vi "Axis Property to Array.vi"(11 "Axis Property In":T2) -> (3 "Axis Property Array Out":T1[](array[typedef]))   [LabVIEW 2020, in "3D Plot.lvclass"]
uses:
  3D Plot.lvclass
  Axis Property.ctl
  Caption Property.ctl
  Label Property.ctl
  Range Property.ctl
  Range Clusters.ctl
  Grid Property.ctl
  Tick Property.ctl
  Axis Property Array Element.ctl
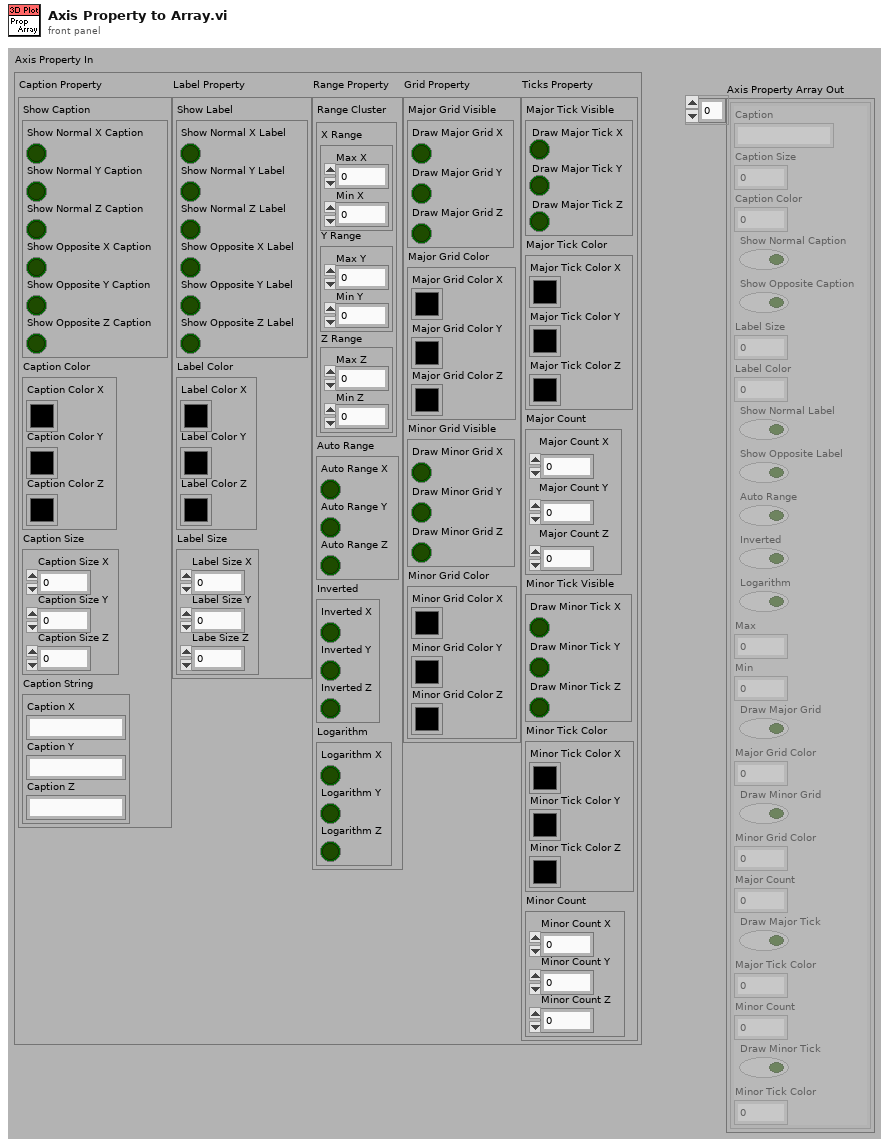
[diagram p1: front panel]
types:
  T1 = typedef "3D Plot.lvclass/Axis Property Array Element.ctl" = cluster{"Caption":string, "Caption Size":u16, "Caption Color":u32, "Show Normal Caption":bool, "Show Opposite Caption":bool, "Label Size":u16, "Label Color":u32, "Show Normal Label":bool, "Show Opposite Label":bool, "Auto Range":bool, "Inverted":bool, "Logarithm":bool, "Max":sgl, "Min":sgl, "Draw Major Grid":bool, "Major Grid Color":u32, "Draw Minor Grid":bool, "Minor Grid Color":u32, "Major Count":u16, "Draw Major Tick":bool, "Major Tick Color":u32, "Minor Count":u16, "Draw Minor Tick":bool, "Minor Tick Color":u32}
  T2 = typedef "3D Plot.lvclass/Axis Property.ctl" = cluster{"Caption Property":T3, "Label Property":T4, "Range Property":T5, "Grid Property":T7, "Ticks Property":T8}
  T3 = typedef "3D Plot.lvclass/Caption Property.ctl" = cluster{"Show Caption":cluster{"Show Normal X Caption":bool, "Show Normal Y Caption":bool, "Show Normal Z Caption":bool, "Show Opposite X Caption":bool, "Show Opposite Y Caption":bool, "Show Opposite Z Caption":bool}, "Caption Color":cluster{"Caption Color X":u32, "Caption Color Y":u32, "Caption Color Z":u32}, "Caption Size":cluster{"Caption Size X":u16, "Caption Size Y":u16, "Caption Size Z":u16}, "Caption String":cluster{"Caption X":string, "Caption Y":string, "Caption Z ":string}}
  T4 = typedef "3D Plot.lvclass/Label Property.ctl" = cluster{"Show Label":cluster{"Show Normal X Label":bool, "Show Normal Y Label":bool, "Show Normal Z Label":bool, "Show Opposite X Label":bool, "Show Opposite Y Label":bool, "Show Opposite Z Label":bool}, "Label Color":cluster{"Label Color X":u32, "Label Color Y":u32, "Label Color Z":u32}, "Label Size":cluster{"Label Size X":u16, "Label Size Y":u16, "Labe Size Z":u16}}
  T5 = typedef "3D Plot.lvclass/Range Property.ctl" = cluster{"Range Cluster":T6, "Auto Range":cluster{"Auto Range X":bool, "Auto Range Y":bool, "Auto Range Z":bool}, "Inverted":cluster{"Inverted X":bool, "Inverted Y":bool, "Inverted Z":bool}, "Logarithm":cluster{"Logarithm X":bool, "Logarithm Y":bool, "Logarithm Z":bool}}
  T6 = typedef "3D Plot.lvclass/Range Clusters.ctl" = cluster{"X Range":cluster{"Max X":sgl, "Min X":sgl}, "Y Range":cluster{"Max Y":sgl, "Min Y":sgl}, "Z Range":cluster{"Max Z":sgl, "Min Z":sgl}}
  T7 = typedef "3D Plot.lvclass/Grid Property.ctl" = cluster{"Major Grid Visible":cluster{"Draw Major Grid X":bool, "Draw Major Grid Y":bool, "Draw Major Grid Z":bool}, "Major Grid Color":cluster{"Major Grid Color X":u32, "Major Grid Color Y":u32, "Major Grid Color Z":u32}, "Minor Grid Visible":cluster{"Draw Minor Grid X":bool, "Draw Minor Grid Y":bool, "Draw Minor Grid Z":bool}, "Minor Grid Color":cluster{"Minor Grid Color X":u32, "Minor Grid Color Y":u32, "Minor Grid Color Z":u32}}
  T8 = typedef "3D Plot.lvclass/Tick Property.ctl" = cluster{"Major Tick Visible":cluster{"Draw Major Tick X":bool, "Draw Major Tick Y":bool, "Draw Major Tick Z":bool}, "Major Tick Color":cluster{"Major Tick Color X":u32, "Major Tick Color Y":u32, "Major Tick Color Z":u32}, "Major Count":cluster{"Major Count X":u16, "Major Count Y":u16, "Major Count Z":u16}, "Minor Tick Visible":cluster{"Draw Minor Tick X":bool, "Draw Minor Tick Y":bool, "Draw Minor Tick Z":bool}, "Minor Tick Color":cluster{"Minor Tick Color X":u32, "Minor Tick Color Y":u32, "Minor Tick Color Z":u32}, "Minor Count":cluster{"Minor Count X":u16, "Minor Count Y":u16, "Minor Count Z":u16}}
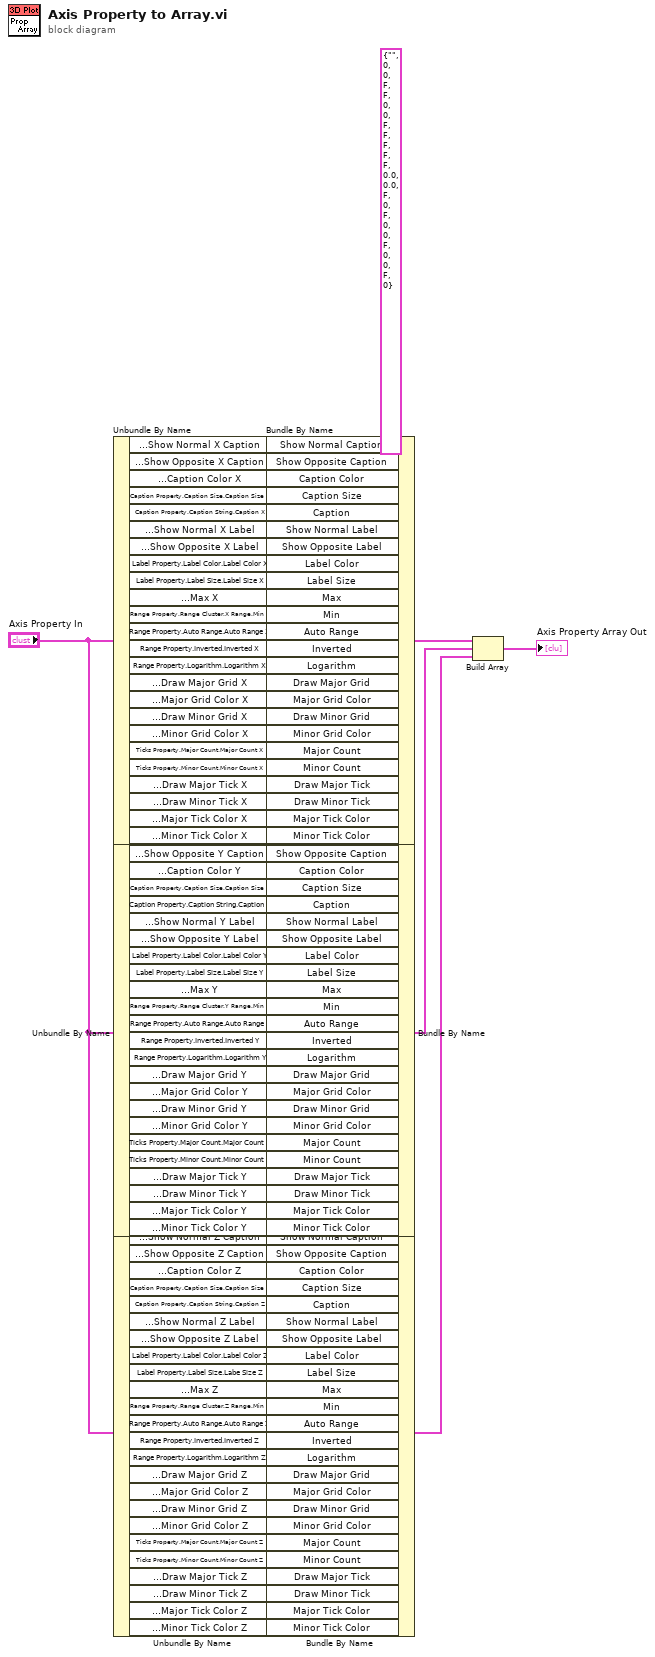
[diagram p0: block diagram]
diagram:
  w6 = T1 {"Caption"="", "Caption Size"=0, "Caption Color"=0, "Show Normal Caption"=FALSE, "Show Opposite Caption"=FALSE, "Label Size"=0, "Label Color"=0, "Show Normal Label"=FALSE, "Show Opposite Label"=FALSE, "Auto Range"=FALSE, "Inverted"=FALSE, "Logarithm"=FALSE, "Max"=0.0, "Min"=0.0, "Draw Major Grid"=FALSE, "Major Grid Color"=0, "Draw Minor Grid"=FALSE, "Minor Grid Color"=0, "Major Count"=0, "Draw Major Tick"=FALSE, "Major Tick Color"=0, "Minor Count"=0, "Draw Minor Tick"=FALSE, "Minor Tick Color"=0} ("output cluster")
  n1 = Unbundle By Name("Axis Property In") -> ("Caption Property.Show Caption.Show Normal X Caption"=w77:bool, "Caption Property.Show Caption.Show Opposite X Caption"=w76:bool, "Caption Property.Caption Color.Caption Color X"=w75:u32, "Caption Property.Caption Size.Caption Size X"=w74:u16, "Caption Property.Caption String.Caption X"=w73:string, "Label Property.Show Label.Show Normal X Label"=w72:bool, "Label Property.Show Label.Show Opposite X Label"=w71:bool, "Label Property.Label Color.Label Color X"=w70:u32, "Label Property.Label Size.Label Size X"=w69:u16, "Range Property.Range Cluster.X Range.Max X"=w68:sgl, "Range Property.Range Cluster.X Range.Min X"=w67:sgl, "Range Property.Auto Range.Auto Range X"=w66:bool, "Range Property.Inverted.Inverted X"=w65:bool, "Range Property.Logarithm.Logarithm X"=w3:bool, "Grid Property.Major Grid Visible.Draw Major Grid X"=w64:bool, "Grid Property.Major Grid Color.Major Grid Color X"=w63:u32, "Grid Property.Minor Grid Visible.Draw Minor Grid X"=w62:bool, "Grid Property.Minor Grid Color.Minor Grid Color X"=w61:u32, "Ticks Property.Major Count.Major Count X"=w60:u16, "Ticks Property.Minor Count.Minor Count X"=w59:u16, "Ticks Property.Major Tick Visible.Draw Major Tick X"=w58:bool, "Ticks Property.Minor Tick Visible.Draw Minor Tick X"=w57:bool, "Ticks Property.Major Tick Color.Major Tick Color X"=w56:u32, "Ticks Property.Minor Tick Color.Minor Tick Color X"=w55:u32)
  n2 = Unbundle By Name("Axis Property In") -> ("Caption Property.Show Caption.Show Normal Y Caption"=w53:bool, "Caption Property.Show Caption.Show Opposite Y Caption"=w52:bool, "Caption Property.Caption Color.Caption Color Y"=w51:u32, "Caption Property.Caption Size.Caption Size Y"=w50:u16, "Caption Property.Caption String.Caption Y"=w49:string, "Label Property.Show Label.Show Normal Y Label"=w48:bool, "Label Property.Show Label.Show Opposite Y Label"=w47:bool, "Label Property.Label Color.Label Color Y"=w46:u32, "Label Property.Label Size.Label Size Y"=w45:u16, "Range Property.Range Cluster.Y Range.Max Y"=w44:sgl, "Range Property.Range Cluster.Y Range.Min Y"=w43:sgl, "Range Property.Auto Range.Auto Range Y"=w42:bool, "Range Property.Inverted.Inverted Y"=w41:bool, "Range Property.Logarithm.Logarithm Y"=w2:bool, "Grid Property.Major Grid Visible.Draw Major Grid Y"=w40:bool, "Grid Property.Major Grid Color.Major Grid Color Y"=w39:u32, "Grid Property.Minor Grid Visible.Draw Minor Grid Y"=w37:bool, "Grid Property.Minor Grid Color.Minor Grid Color Y"=w36:u32, "Ticks Property.Major Count.Major Count Y"=w35:u16, "Ticks Property.Minor Count.Minor Count Y"=w34:u16, "Ticks Property.Major Tick Visible.Draw Major Tick Y"=w33:bool, "Ticks Property.Minor Tick Visible.Draw Minor Tick Y"=w32:bool, "Ticks Property.Major Tick Color.Major Tick Color Y"=w31:u32, "Ticks Property.Minor Tick Color.Minor Tick Color Y"=w30:u32)
  n3 = Unbundle By Name("Axis Property In") -> ("Caption Property.Show Caption.Show Normal Z Caption"=w29:bool, "Caption Property.Show Caption.Show Opposite Z Caption"=w28:bool, "Caption Property.Caption Color.Caption Color Z"=w27:u32, "Caption Property.Caption Size.Caption Size Z"=w26:u16, "Caption Property.Caption String.Caption Z"=w25:string, "Label Property.Show Label.Show Normal Z Label"=w24:bool, "Label Property.Show Label.Show Opposite Z Label"=w23:bool, "Label Property.Label Color.Label Color Z"=w22:u32, "Label Property.Label Size.Labe Size Z"=w21:u16, "Range Property.Range Cluster.Z Range.Max Z"=w20:sgl, "Range Property.Range Cluster.Z Range.Min Z"=w19:sgl, "Range Property.Auto Range.Auto Range Z"=w18:bool, "Range Property.Inverted.Inverted Z"=w17:bool, "Range Property.Logarithm.Logarithm Z"=w1:bool, "Grid Property.Major Grid Visible.Draw Major Grid Z"=w16:bool, "Grid Property.Major Grid Color.Major Grid Color Z"=w15:u32, "Grid Property.Minor Grid Visible.Draw Minor Grid Z"=w14:bool, "Grid Property.Minor Grid Color.Minor Grid Color Z"=w13:u32, "Ticks Property.Major Count.Major Count Z"=w12:u16, "Ticks Property.Minor Count.Minor Count Z"=w11:u16, "Ticks Property.Major Tick Visible.Draw Major Tick Z"=w10:bool, "Ticks Property.Minor Tick Visible.Draw Minor Tick Z"=w9:bool, "Ticks Property.Major Tick Color.Major Tick Color Z"=w8:u32, "Ticks Property.Minor Tick Color.Minor Tick Color Z"=w7:u32)
  n4 = Bundle By Name(cluster=w6, "Show Normal Caption"=w77, "Show Opposite Caption"=w76, "Caption Color"=w75, "Caption Size"=w74, "Caption"=w73, "Show Normal Label"=w72, "Show Opposite Label"=w71, "Label Color"=w70, "Label Size"=w69, "Max"=w68, "Min"=w67, "Auto Range"=w66, "Inverted"=w65, "Logarithm"=w3, "Draw Major Grid"=w64, "Major Grid Color"=w63, "Draw Minor Grid"=w62, "Minor Grid Color"=w61, "Major Count"=w60, "Minor Count"=w59, "Draw Major Tick"=w58, "Draw Minor Tick"=w57, "Major Tick Color"=w56, "Minor Tick Color"=w55) -> (w54:T1)
  n5 = Bundle By Name(cluster=w6, "Show Normal Caption"=w53, "Show Opposite Caption"=w52, "Caption Color"=w51, "Caption Size"=w50, "Caption"=w49, "Show Normal Label"=w48, "Show Opposite Label"=w47, "Label Color"=w46, "Label Size"=w45, "Max"=w44, "Min"=w43, "Auto Range"=w42, "Inverted"=w41, "Logarithm"=w2, "Draw Major Grid"=w40, "Major Grid Color"=w39, "Draw Minor Grid"=w37, "Minor Grid Color"=w36, "Major Count"=w35, "Minor Count"=w34, "Draw Major Tick"=w33, "Draw Minor Tick"=w32, "Major Tick Color"=w31, "Minor Tick Color"=w30) -> (w38:T1)
  n6 = Bundle By Name(cluster=w6, "Show Normal Caption"=w29, "Show Opposite Caption"=w28, "Caption Color"=w27, "Caption Size"=w26, "Caption"=w25, "Show Normal Label"=w24, "Show Opposite Label"=w23, "Label Color"=w22, "Label Size"=w21, "Max"=w20, "Min"=w19, "Auto Range"=w18, "Inverted"=w17, "Logarithm"=w1, "Draw Major Grid"=w16, "Major Grid Color"=w15, "Draw Minor Grid"=w14, "Minor Grid Color"=w13, "Major Count"=w12, "Minor Count"=w11, "Draw Major Tick"=w10, "Draw Minor Tick"=w9, "Major Tick Color"=w8, "Minor Tick Color"=w7) -> (w5:T1)
  n7 = Build Array(w54, w38, w5) -> (→"Axis Property Array Out":T1[])
